vi "Pre-Build Action.vi"(6 "Top Level/Always Included VIs":path[](array[path]), 7 "Main Destination Path":path, 9 "Target Name":string, 10 "Build Specification Name":string, 11 "Project Path":path) -> (0 "error out":errorcluster)   [LabVIEW 2018]
uses:
  <vilib>/Utility/config.llb/Write Key (String).vi
  <vilib>/Utility/config.llb/NI_LVConfig.lvlib
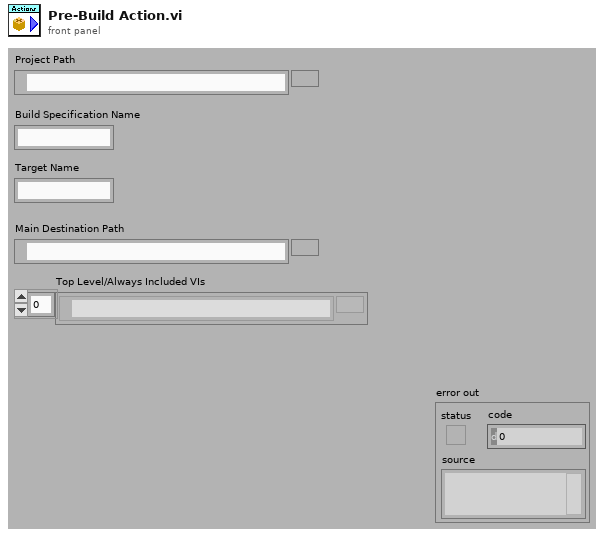
[diagram p1: front panel]
types:
  T1 = enum16{"open", "replace", "create", "open or create", "replace or create", "replace or create with confirmation"}
  T2 = typedef "NI_LVConfig.lvlib/Config Data RefNum.ctl" = refnum<k1>
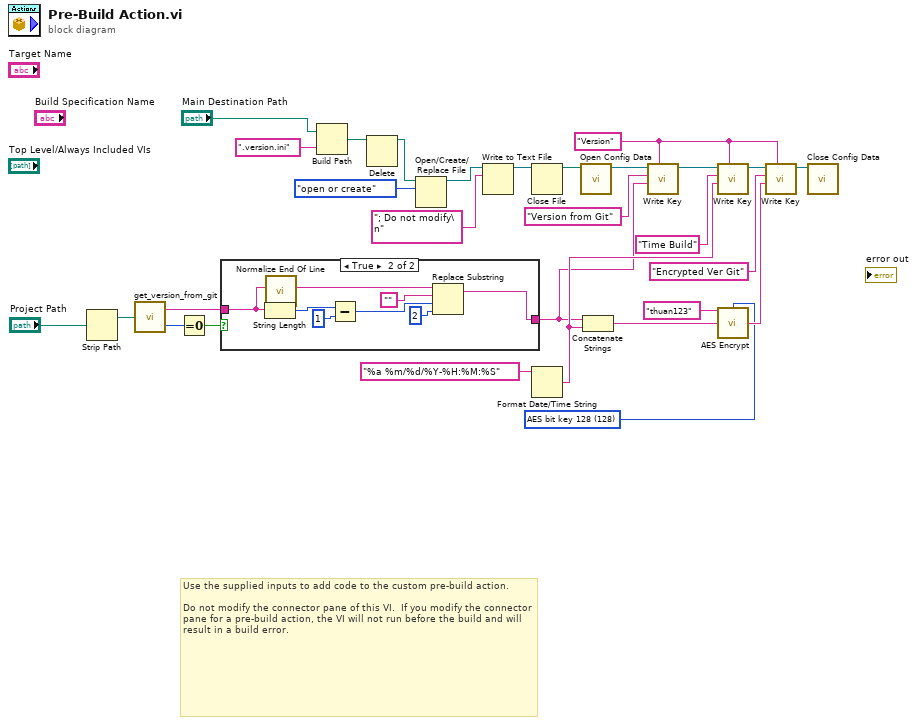
[diagram p0: block diagram]
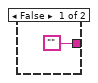
[diagram p2: hidden frame]
diagram:
  w9 = u16 128 items=["AES bit key 128"=128, "AES bit key 192"=192, "AES bit key 256"=256] ("BitKeyType(256)")
  w6 = "Version" ("key")
  # "Use the supplied inputs to add code to the custom pre-build action.\n\nDo not modify the connector pane of this VI.  If you modify the connector pane for a pre-build action, the VI will not run before the build and will result in a build error."
  n1 = Strip Path(path="Project Path") -> (stripped path=w28:path)  [unwired: 1 out]
  n2 = call "get_version_from_git.vi"("path_project"=w28) -> ("Version"=w23:string, "return code"=w22:i32)
  n3 = Equal To 0?(x=w22) -> (x = 0?=w21:bool)
  n4 = case shown="True" w21 {
    tunnel: ["" w37] -> w2
    tunnel: w23 -> [_ w35]
    frame False {
    }
    frame True {
      n5 = String Length(string=w35) -> (length=w34:i32)
      n6 = call <vilib>:"Normalize End Of Line.vi"("string in"=w35) -> ("string out"=w38:string)  [unwired: 7 in]
      n7 = Subtract(x=w34, y=1) -> (x-y=w32:i32)
      n8 = Replace Substring(2:2 ("length (len. of substring)"), 3:w32, 4:"", 5:w38) -> (1:w37:string)  [unwired: 1 out]
    }
  }
  n9 = Build Path(base path="Main Destination Path", name or relative path=".version.ini") -> (appended path=w25:path)
  n10 = Delete(path (use dialog)=w25) -> (deleted path=w20:path)  [unwired: 4 in, 2 out]
  n11 = Open/Create/Replace File(file path (use dialog)=w20, operation (0:open)=T1."open or create") -> (refnum out=w18:refnum<file>)  [unwired: 4 in, 2 out]
  n12 = Write to Text File(file (use dialog)=w18, text="; Do not modify\n") -> (refnum out=w16:refnum<file>)  [unwired: 2 in, 2 out]
  n13 = Close File(refnum=w16) -> (path=w14:path)  [unwired: 1 in, 1 out]
  n14 = Format Date/Time String(time format string (%c)="%a %m/%d/%Y-%H:%M:%S") -> (date/time string=w3:string)  [unwired: 2 in]
  n15 = call <vilib>:"Open Config Data.vi"("configuration file path"=w14) -> ("refnum"=w15:T2)  [unwired: 2 in, 8 out]
  n16 = Concatenate Strings(w2, w3) -> (w1:string)
  n17 = call-poly <vilib>:"Write Key.vi"("section"=w6, "value"=w2, "key"="Version from Git", "refnum"=w15) -> ("refnum out"=w8:T2)  [unwired: 5 in, 2 out]
  n18 = call-poly <vilib>:"Write Key.vi"("section"=w6, "value"=w3, "key"="Time Build", "refnum"=w8) -> ("refnum out"=w7:T2)  [unwired: 5 in, 2 out]
  n19 = call "AES Encrypt.vi"("Password.In"="thuan123", "BitKeyType(256)"=w9, "PlainText.In"=w1) -> ("CypheredText out"=w12:string)  [unwired: 11 in, 1 out]
  n20 = call-poly <vilib>:"Write Key.vi"("section"=w6, "value"=w12, "key"="Encrypted Ver Git", "refnum"=w7) -> ("refnum out"=w10:T2)  [unwired: 5 in, 2 out]
  n21 = call <vilib>:"Close Config Data.vi"("refnum"=w10) -> ()  [unwired: 9 in, 2 out]
